vi "Generate Profile.vi"(8 "error in (no error)":errorcluster, 11 "EIS Parameters":T1 {"EIS Mode" items=["Voltage (PEIS)"=1, "Current (GEIS)"=2]}) -> (0 "error out":errorcluster, 1 "EIS Profile":waveform(dbl)[](array[waveform]), 2 "Voltage Profile out":waveform(dbl)[](array[waveform]), 3 "Current Profile out":waveform(dbl)[](array[waveform]), 5 "Frequencies":dbl[](array[numeric]))   [LabVIEW 2023, in "ACIR_EIS.lvclass"]
uses:
  ACIR_EIS.lvclass
  Types/EIS Parameters.ctl
  Types/EIS Mode.ctl
  <vilib>/Waveform/WDTOps.llb/WDT Append Waveforms DBL.vi
  ACIR_EIS.lvclass/ACIR_EIS.ctl
  <vilib>/measure/NI_MABase.lvlib
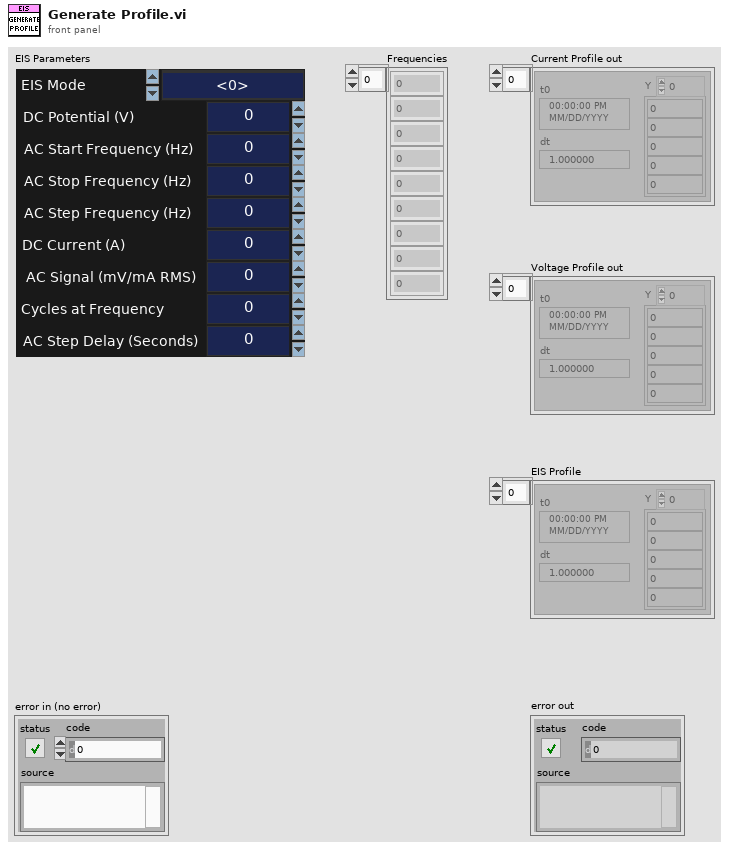
[diagram p1: front panel]
types:
  T1 = typedef "EIS Parameters.ctl" = cluster{"EIS Mode":T2, "EIS DC Potential":dbl, "EIS Start Frequency":dbl, "EIS Stop Frequency":dbl, "EIS Delta Frequency":dbl, "EIS DC Current":dbl, "AC Signal (mV/mA RMS)":dbl, "Cycles at Frequency":dbl, "EIS AC Step Delay":dbl}
  T2 = typedef "EIS Mode.ctl" = u16
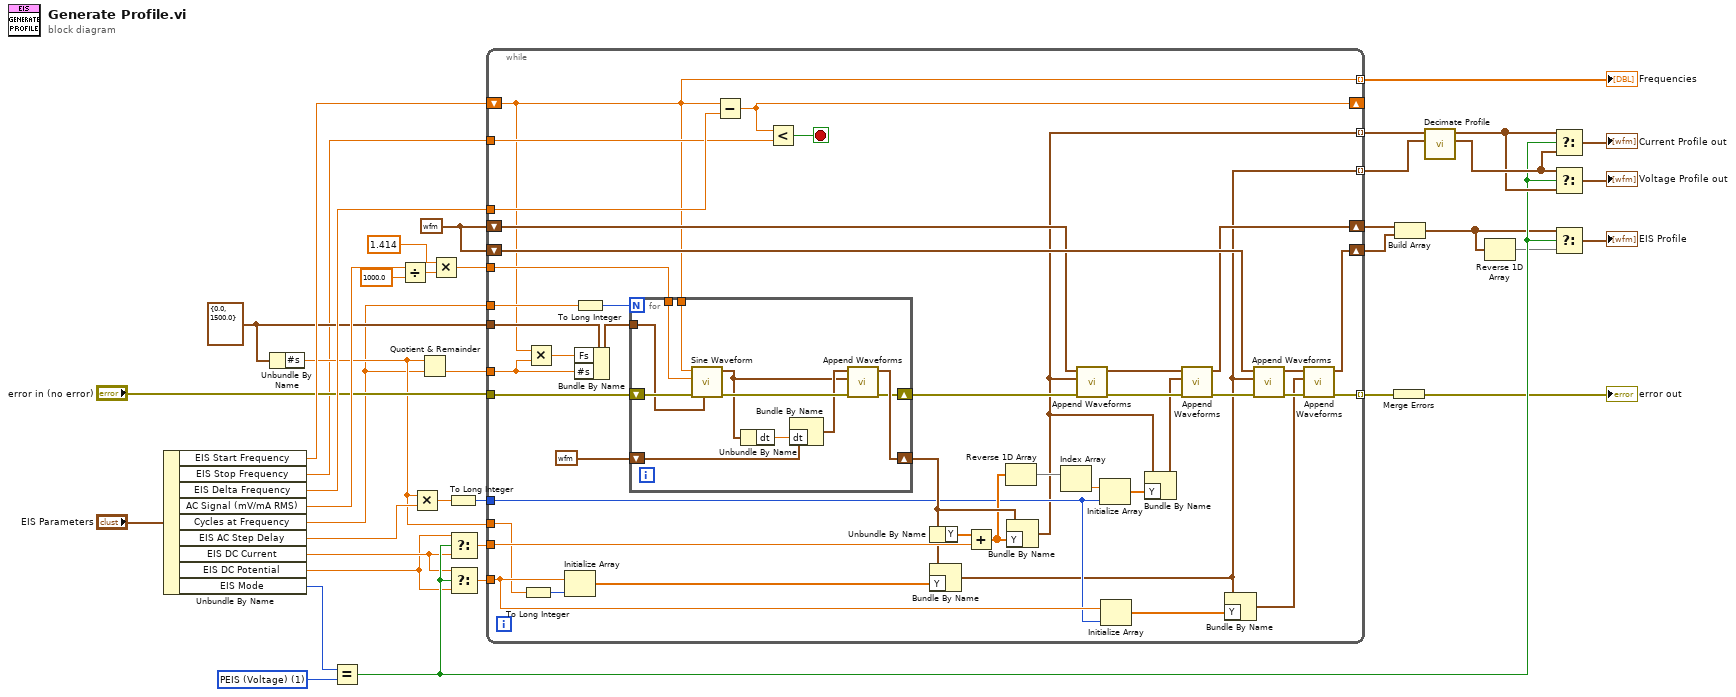
[diagram p0: block diagram]
diagram:
  w12 = waveform(dbl) {"t0"=timestamp(0 s since 1904-01-01), "dt"=1.0, "Y"=[]} ("waveform out")
  w6 = cluster{"Fs":dbl, "#s":dbl} {"Fs"=0.0, "#s"=1500.0} ("EIS Sampling Info")
  w9 = T2 1 items=["PEIS (Voltage)"=1, "GEIS (Current)"=2] ("x")
  n1 = Unbundle By Name("EIS Parameters") -> ("EIS Start Frequency"=w28:dbl, "EIS Stop Frequency"=w2:dbl, "EIS Delta Frequency"=w27:dbl, "AC Signal (mV/mA RMS)"=w26:dbl, "Cycles at Frequency"=w4:dbl, "EIS AC Step Delay"=w34:dbl, "EIS DC Current"=w25:dbl, "EIS DC Potential"=w24:dbl, "EIS Mode"=w29:T2)
  n2 = Unbundle By Name(w6) -> ("#s"=w5:dbl)
  n3 = Equal?(x=w29, y=w9) -> (x = y?=w31:bool)
  n4 = Divide(x=w26, y=1000.0) -> (x/y=w18:dbl)
  n5 = Multiply(x=w5, y=w34) -> (x*y=w20:dbl)
  n6 = Quotient & Remainder(x=w5, y=w4) -> (floor(x/y)=w3:dbl)  [unwired: 1 out]
  n7 = Multiply(x=1.414, y=w18) -> (x*y=w19:dbl)
  n8 = To Long Integer(number=w20) -> (32bit integer=w21:i32)
  n9 = Select(t=w24, s=w31, f=w25) -> (s? t:f=w17:dbl)
  n10 = Select(t=w25, s=w31, f=w24) -> (s? t:f=w16:dbl)
  n11 = while {
    tunnel: w17 -> [w78]
    tunnel: w27 -> [w81]
    shift-right: [w43] -> _
    shift-left: w28 -> [w40]
    tunnel: [w69] -> w10 mode=indexing
    tunnel: "error in (no error)" -> [w80]
    tunnel: w19 -> [w79]
    tunnel: w16 -> [w64]
    shift-right: [w55] -> w23
    shift-left: w12 -> [w58]
    shift-right: [w57] -> w22
    shift-left: w12 -> [w74]
    tunnel: w21 -> [w61]
    tunnel: w5 -> [w46]
    tunnel: [w53] -> w35 mode=indexing
    tunnel: [w52] -> w36 mode=indexing
    tunnel: w6 -> [w48]
    tunnel: w4 -> [w51]
    tunnel: w3 -> [w45]
    tunnel: w2 -> [w42]
    tunnel: [w40] -> w1 mode=indexing
    stop <- w41 stop-if-true
    n12 = To Long Integer(number=w46) -> (32bit integer=w63:i32)
    n13 = Multiply(x=w40, y=w45) -> (x*y=w49:dbl)
    n14 = Initialize Array(w64, w63) -> (w77:dbl[])
    n15 = To Long Integer(number=w51) -> (32bit integer=w50:i32)
    n16 = Bundle By Name(cluster=w48, "Fs"=w49, "#s"=w45) -> (w47:cluster{"Fs":dbl, "#s":dbl})
    n17 = for {
      N: w50 -> [_]
      tunnel: w79 -> [w91]
      tunnel: w40 -> [w90]
      tunnel: w47 -> [w88]
      shift-right: [w86] -> w75
      shift-left: w80 -> [w92]
      shift-right: [w89] -> w73
      shift-left: waveform(dbl) {"t0"=timestamp(0 s since 1904-01-01), "dt"=1.0, "Y"=[]} ("waveform out") -> [w85]
      n18 = call <vilib>:"Sine Waveform.vi"("sampling info"=w88, "error in (no error)"=w92, "amplitude"=w91, "frequency"=w90) -> ("error out"=w87:errorcluster, "signal out"=w82:waveform(dbl))  [unwired: 6 in]
      n19 = Unbundle By Name(w82) -> ("dt"=w84:dbl)
      n20 = Bundle By Name(cluster=w85, "dt"=w84) -> (w83:waveform(dbl))
      n21 = call-poly <vilib>:"Append Waveforms.vi"("error in (no error)"=w87, "waveform B"=w82, "waveform A"=w83) -> ("error out"=w86:errorcluster, "waveform out"=w89:waveform(dbl))  [unwired: 7 in]
    }
    n22 = Subtract(x=w40, y=w81) -> (x-y=w43:dbl)
    n23 = Less?(x=w43, y=w42) -> (x < y?=w41:bool)
    n24 = Unbundle By Name(w73) -> ("Y"=w76:dbl[])
    n25 = Bundle By Name(cluster=w73, "Y"=w77) -> (w52:waveform(dbl))
    n26 = Add(x=w76, y=w78) -> (x+y=w68:dbl[])
    n27 = Reverse 1D Array(array=w68) -> (reversed array=w67:dbl[])
    n28 = Bundle By Name(cluster=w73, "Y"=w68) -> (w53:waveform(dbl))
    n29 = Index Array(array=w67) -> (element=w66:dbl)  [unwired: 1 in]
    n30 = call-poly <vilib>:"Append Waveforms.vi"("error in (no error)"=w75, "waveform B"=w53, "waveform A"=w58) -> ("error out"=w72:errorcluster, "waveform out"=w56:waveform(dbl))  [unwired: 7 in]
    n31 = Initialize Array(w66, w61) -> (w65:dbl[])
    n32 = Initialize Array(w64, w61) -> (w60:dbl[])
    n33 = Bundle By Name(cluster=w53, "Y"=w65) -> (w62:waveform(dbl))
    n34 = call-poly <vilib>:"Append Waveforms.vi"("error in (no error)"=w72, "waveform B"=w62, "waveform A"=w56) -> ("error out"=w71:errorcluster, "waveform out"=w55:waveform(dbl))  [unwired: 7 in]
    n35 = Bundle By Name(cluster=w52, "Y"=w60) -> (w59:waveform(dbl))
    n36 = call-poly <vilib>:"Append Waveforms.vi"("error in (no error)"=w71, "waveform B"=w52, "waveform A"=w74) -> ("error out"=w70:errorcluster, "waveform out"=w54:waveform(dbl))  [unwired: 7 in]
    n37 = call-poly <vilib>:"Append Waveforms.vi"("error in (no error)"=w70, "waveform B"=w59, "waveform A"=w54) -> ("error out"=w69:errorcluster, "waveform out"=w57:waveform(dbl))  [unwired: 7 in]
  }
  "Frequencies" <- w1
  n38 = Merge Errors(w10) -> (→"error out":errorcluster)
  n39 = Build Array(w23, w22) -> (w13:waveform(dbl)[])
  n40 = call "Decimate Profile.vi"("Current Profile in"=w36, "Voltage Profile in"=w35) -> ("Current Profile out"=w38:waveform(dbl)[], "Voltage Profile out"=w37:waveform(dbl)[])  [unwired: 8 in]
  n41 = Reverse 1D Array(array=w13) -> (reversed array=w14:waveform(dbl)[])
  n42 = Select(t=w37, s=w31, f=w38) -> (s? t:f=→"Current Profile out":waveform(dbl)[])
  n43 = Select(t=w38, s=w31, f=w37) -> (s? t:f=→"Voltage Profile out":waveform(dbl)[])
  n44 = Select(t=w13, s=w31, f=w14) -> (s? t:f=→"EIS Profile":waveform(dbl)[])
